vi "Read Chirp Frequency Ends(Hz)V2.vi"(8 "error in (no error)":errorcluster, 11 "ChirpV2 in":refnum<class "ChirpV2.lvclass">) -> (0 "error out":errorcluster, 2 "Chirp Frequency Ends(Hz)":dbl, 3 "ChirpV2 out":refnum<class "ChirpV2.lvclass">)   [LabVIEW 2014, in "ChirpV2.lvclass"]
uses:
  ChirpV2.lvclass
  ChirpV2.lvclass/ChirpV2.ctl
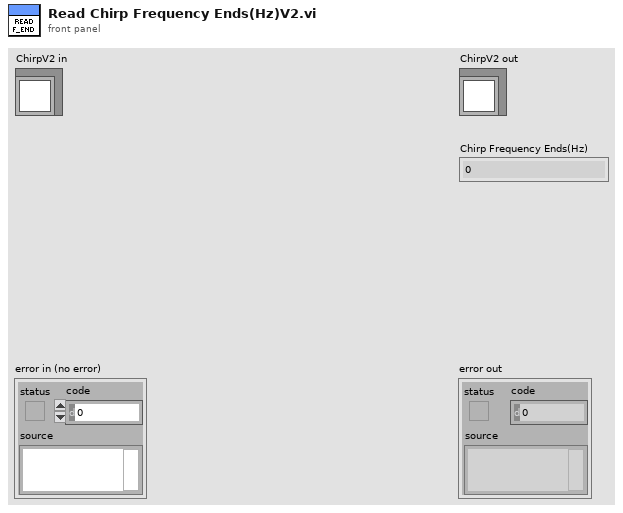
[diagram p1: front panel]
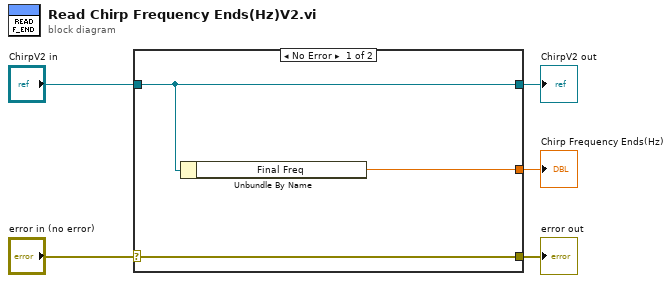
[diagram p0: block diagram]
diagram:
  n1 = case shown="No Error" "error in (no error)" {
    selector: "error in (no error)" -> [w8 w9]
    tunnel: [w8 w9] -> w4
    tunnel: [w7 w10] -> w2
    tunnel: "ChirpV2 in" -> [w7 w10]
    tunnel: [w6 _] -> w1
    frame No Error {
      n2 = Unbundle By Name(w7) -> ("Final Freq"=w6:dbl)
    }
    frame Error {
    }
  }
  "error out" <- w4
  "ChirpV2 out" <- w2
  "Chirp Frequency Ends(Hz)" <- w1
